vi "NtoFPGA.vi"(3 "error in":errorcluster, 5 "number":i32) -> (0 "error out":errorcluster)   [LabVIEW 2013]
uses:
  <vilib>/DAQmx/write.llb/DAQmx Write (Digital Bool 1Line 1Point).vi
  <vilib>/DAQmx/miscellaneous.llb/DAQmx Fill In Error Info.vi
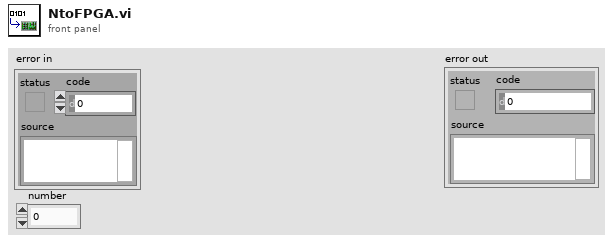
[diagram p1: front panel]
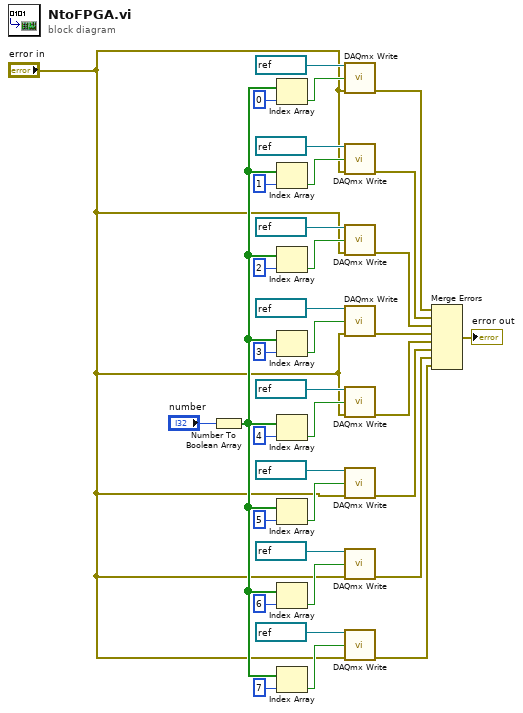
[diagram p0: block diagram]
diagram:
  n1 = Number To Boolean Array(number="number") -> (Boolean array=w16:bool[])
  n2 = Index Array(array=w16, index=0) -> (element=w31:bool)
  n3 = Index Array(array=w16, index=1) -> (element=w30:bool)
  n4 = Index Array(array=w16, index=2) -> (element=w29:bool)
  n5 = Index Array(array=w16, index=3) -> (element=w28:bool)
  n6 = Index Array(array=w16, index=4) -> (element=w27:bool)
  n7 = Index Array(array=w16, index=5) -> (element=w10:bool)
  n8 = Index Array(array=w16, index=6) -> (element=w11:bool)
  n9 = Index Array(array=w16, index=7) -> (element=w12:bool)
  n10 = call-poly <vilib>:"DAQmx Write.vi"("task/channels in"=refnum<k21> "BIT1", "data"=w31, "error in"="error in") -> ("error out"=w26:errorcluster)  [unwired: 10 in, 2 out]
  n11 = call-poly <vilib>:"DAQmx Write.vi"("task/channels in"=refnum<k21> "BIT2", "data"=w30, "error in"="error in") -> ("error out"=w25:errorcluster)  [unwired: 10 in, 2 out]
  n12 = call-poly <vilib>:"DAQmx Write.vi"("task/channels in"=refnum<k21> "BIT3", "data"=w29, "error in"="error in") -> ("error out"=w24:errorcluster)  [unwired: 10 in, 2 out]
  n13 = call-poly <vilib>:"DAQmx Write.vi"("task/channels in"=refnum<k21> "BIT4", "data"=w28, "error in"="error in") -> ("error out"=w23:errorcluster)  [unwired: 10 in, 2 out]
  n14 = call-poly <vilib>:"DAQmx Write.vi"("task/channels in"=refnum<k21> "BIT5", "data"=w27, "error in"="error in") -> ("error out"=w22:errorcluster)  [unwired: 10 in, 2 out]
  n15 = call-poly <vilib>:"DAQmx Write.vi"("task/channels in"=refnum<k21> "BIT6", "data"=w10, "error in"="error in") -> ("error out"=w9:errorcluster)  [unwired: 10 in, 2 out]
  n16 = call-poly <vilib>:"DAQmx Write.vi"("task/channels in"=refnum<k21> "BIT7", "data"=w11, "error in"="error in") -> ("error out"=w8:errorcluster)  [unwired: 10 in, 2 out]
  n17 = call-poly <vilib>:"DAQmx Write.vi"("task/channels in"=refnum<k21> "BIT8", "data"=w12, "error in"="error in") -> ("error out"=w7:errorcluster)  [unwired: 10 in, 2 out]
  n18 = Merge Errors(w26, w25, w24, w23, w22, w9, w8, w7) -> (→"error out":errorcluster)
